vi "PrepRunDiluteExt_v01.vi"(2 "Debug Mode":bool, 3 "Elapsed Time(s)":dbl, 4 "State":enum16{"Edit", "Start", "Run", "End", "Idle"}(ring), 5 "Argument List In":string[](array[string])) -> (0 "Status Out":string, 1 "Argument List Out":string[](array[string]))   [LabVIEW 2011]
panel:
  in  "Pbub Prep":bool caption="Pre-run"
  out "Pbub Prep var":bool
  out "Pbub?":bool
  in  "Pbub Flow":dbl caption="P bubbler Flow (0-100 sccm)" format="%.2f"
  in  "Pbub Run":bool caption="Run"
  out "GAMFC3 var":dbl=100.0 caption="R3 (0-1000 sscm)" format="%.1f"
  out "GAMFC2 var":dbl=10.0 caption="R2 (0-100 sscm)" format="%.2f"
  out "GAMFC1 var":dbl caption="R1 (0-10 sscm)" format="%.2f"
  out "Ga Flow var":dbl caption="Ga Flow (0-10 sscm)" format="%.4f"
  out "In Prep var":bool
  out "Ga Prep var":bool
  out "Al Prep var":bool
  out "PH3 Prep var":bool
  out "AsH3 Prep var":bool
  out "prep_done":bool
  out "run started":bool
  out "first":bool=TRUE
  out "total time":dbl
  out "is OK?":bool
  out "AsH3?":bool
  out "PH3?":bool
  out "In?":bool
  out "Ga?":bool
  out "Al?":bool
  in  "AsH3 Prep":bool caption="Pre-run"
  in  "PH3 Prep":bool caption="Pre-run"
  in  "In Prep":bool caption="Pre-run"
  in  "prep_time":dbl caption="pre-run time (s)"
  in  "Al Prep":bool caption="Pre-run"
  in  "AsH3 Run":bool caption="Run"
  in  "AsH3 Flow":dbl caption="AsH3 Flow (0-10 sccm)" format="%.2f"
  in  "PH3 Flow":dbl caption="PH3 Flow (0-100 sccm)" format="%.2f"
  in  "PH3 Run":bool caption="Run"
  in  "In Flow":dbl caption="In Flow (0-100 sscm)" format="%.2f"
  in  "In Run":bool caption="Run"
  in  "Al Run":bool caption="Run"
  in  "Al Flow":dbl caption="Al Flow (0-100 sscm)" format="%.2f"
  in  "Cancel":bool
  in  "OK":bool
  out "tTotal(s) 2":dbl
  in  "Ga Tab Control":enum32{"Page 1", "Page 2", "Page 3"}(tab)
  in  "Ga Dilution":bool caption="Dilute"
  in  "Ga Run":bool caption="Run"
  in  "Ga Prep":bool caption="Pre-run"
  out "Ga Flow val":dbl=1.0 caption="Ga Flow (0-10 sscm)" format="%.4f"
  in  "Ga Flow set":dbl caption="Ga Flow (0-10 sscm)" format="%.4f"
  out "GAMFC1 val":dbl caption="R1 (0-10 sscm)" format="%.4f"
  out "GAMFC3 val":dbl=100.0 caption="R3 (0-1000 sscm)" format="%.1f"
  out "GAMFC2 val":dbl=10.0 caption="R2 (0-100 sscm)" format="%.2f"
  in  "GAMFC1 set":dbl=1.0 caption="R1 (0-10 sscm)" format="%.2f"
  in  "GAMFC2 set":dbl=10.0 caption="R2 (0-100 sscm)" format="%.2f"
  in  "GAMFC3 set":dbl=100.0 caption="R3 (0-1000 sscm)" format="%.1f"
  in  "Ga Calculated":u16(ring)=1 caption="Calculated" items=["Ga flow", "MFC1", "MFC2", "MFC3"]
  # "Add pre-run time to run time in editor."
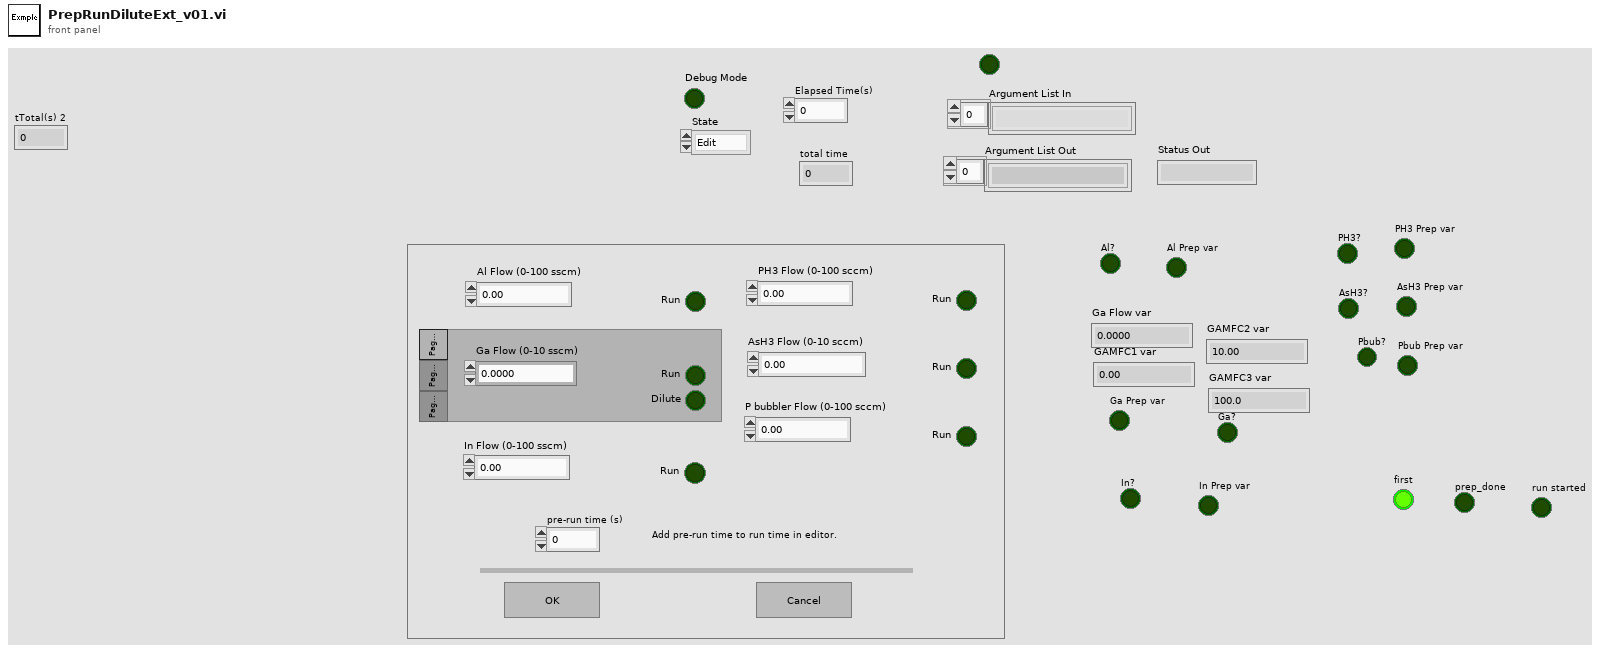
[diagram p1: front panel]
types:
  T1 = enum16{"Discrete", "Continuous", "Instantaneous", "Finite"}
  T2 = enum32{"Invalid", "Default", "Floating", "Floating/Auto-Hide", "Modal"}
  T3 = cluster{"Ga val":bool, "MFC1 val":bool, "MFC2 val":bool, "MFC3 val":bool, "Ga set":bool, "MFC1 set":bool, "MFC2 set":bool, "MFC3 set":bool}
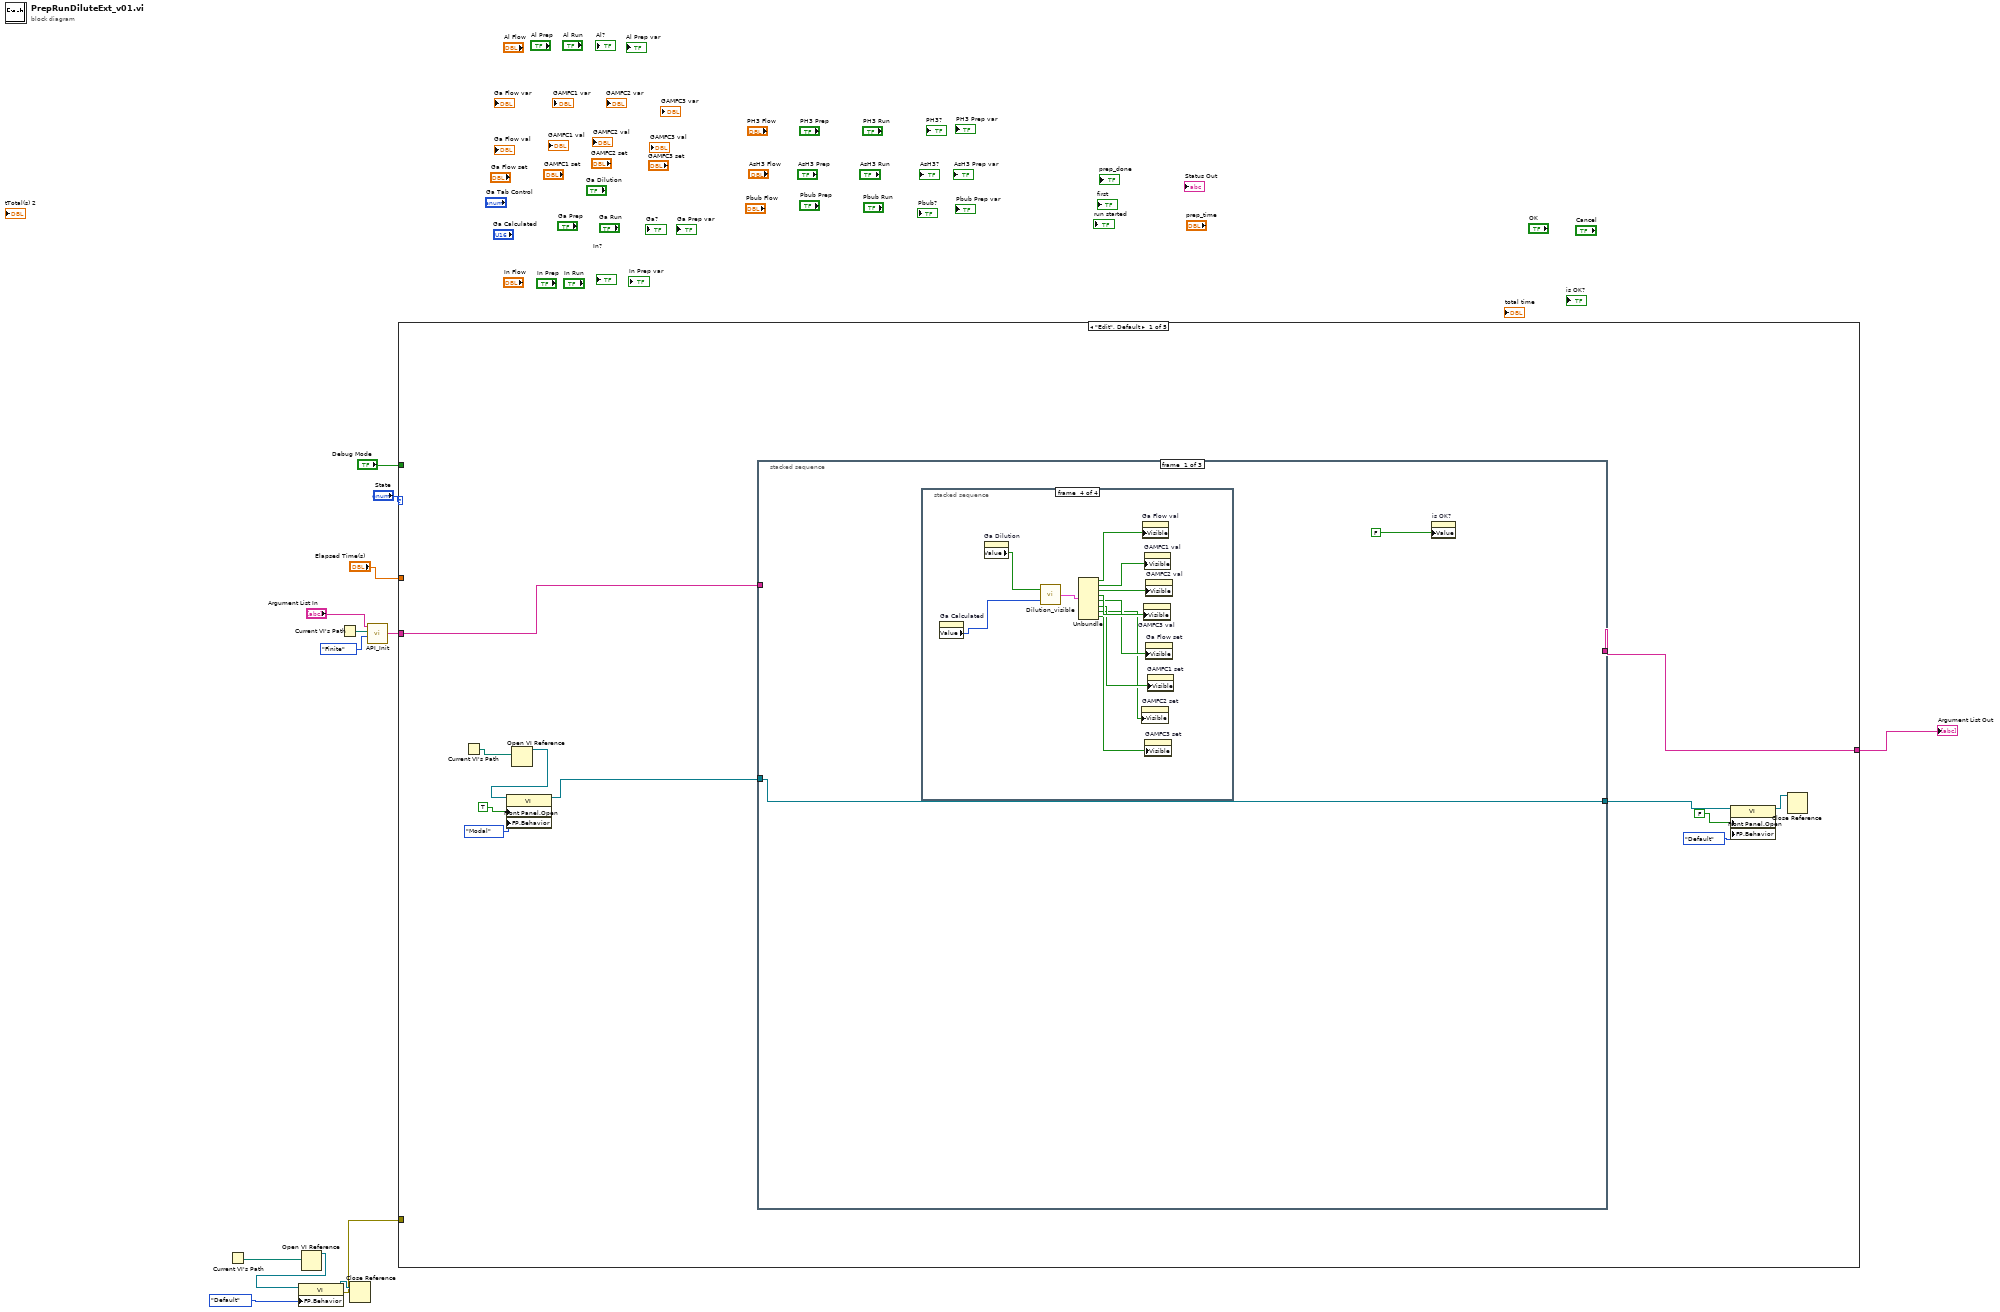
[diagram p0: block diagram]
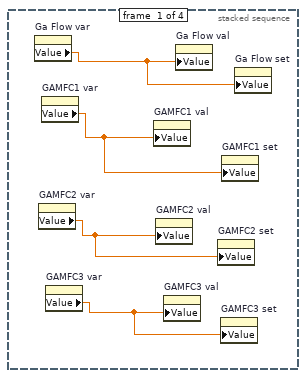
[diagram p2: hidden frame]
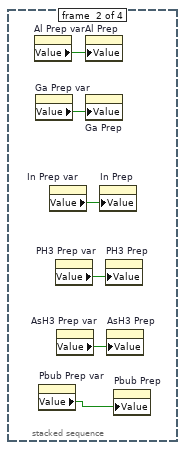
[diagram p3: hidden frame]
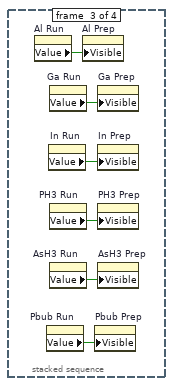
[diagram p4: hidden frame]
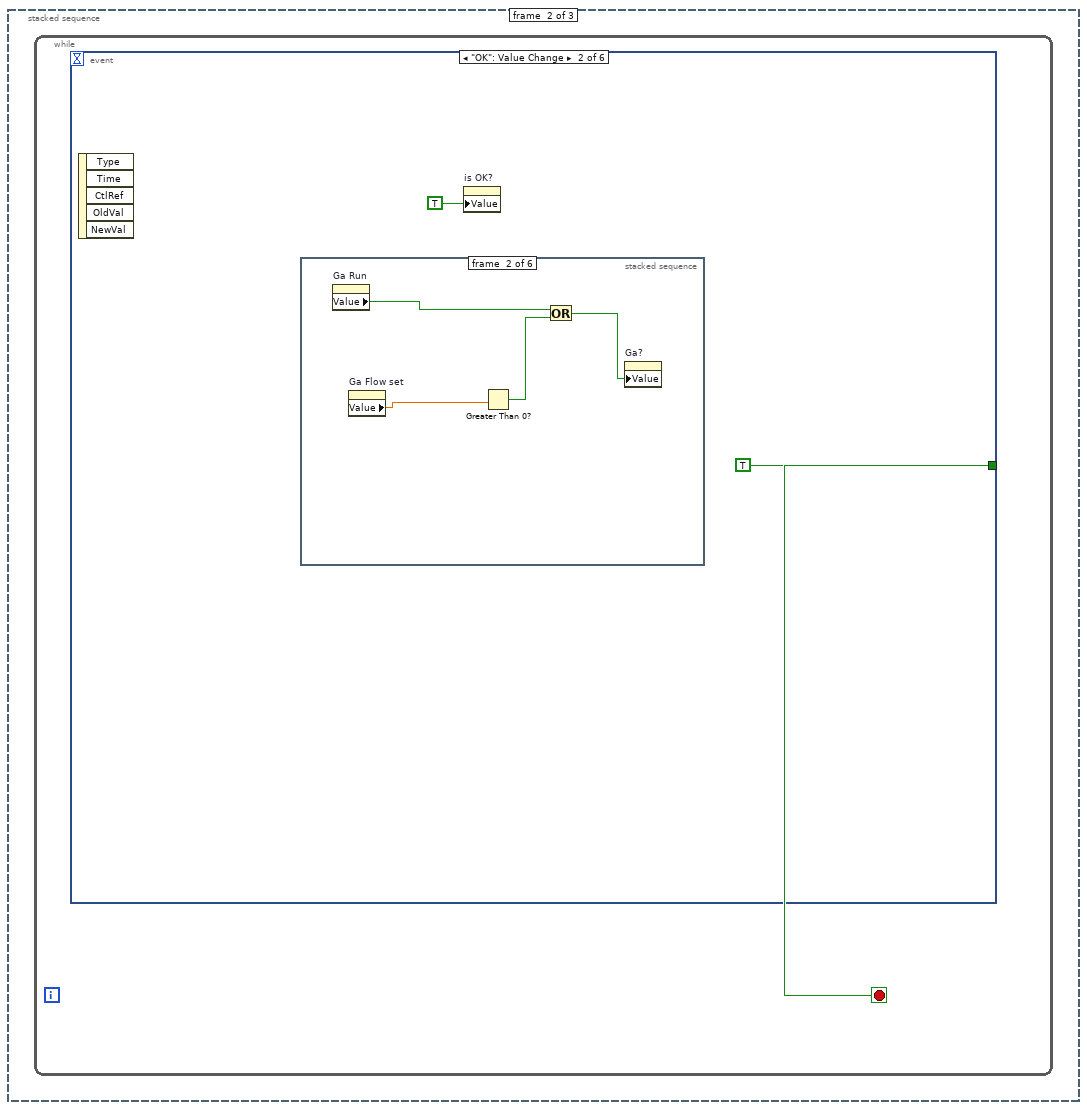
[diagram p5: hidden frame]
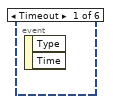
[diagram p6: hidden frame]
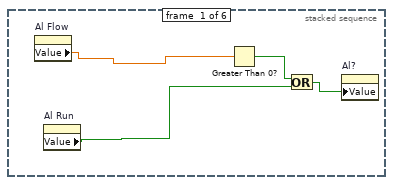
[diagram p7: hidden frame]
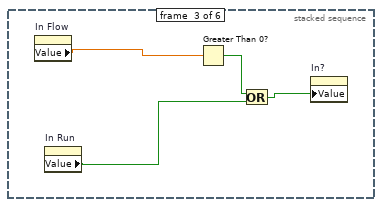
[diagram p8: hidden frame]
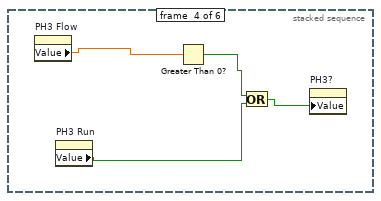
[diagram p9: hidden frame]
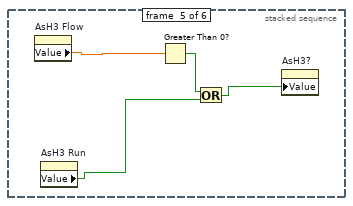
[diagram p10: hidden frame]
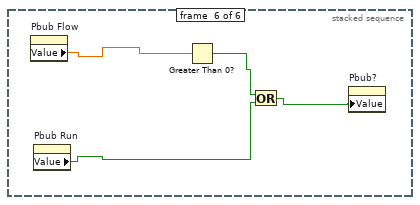
[diagram p11: hidden frame]
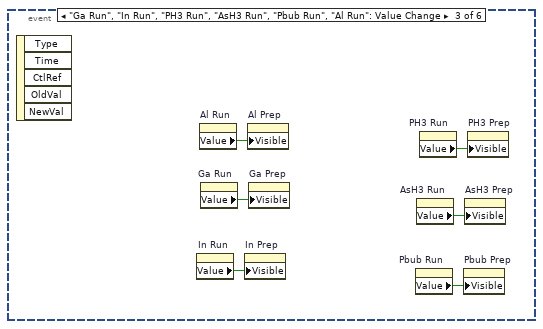
[diagram p12: hidden frame]
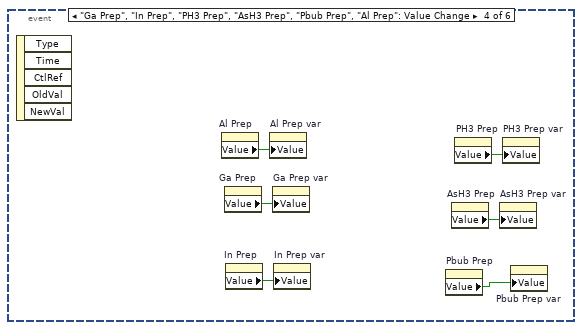
[diagram p13: hidden frame]
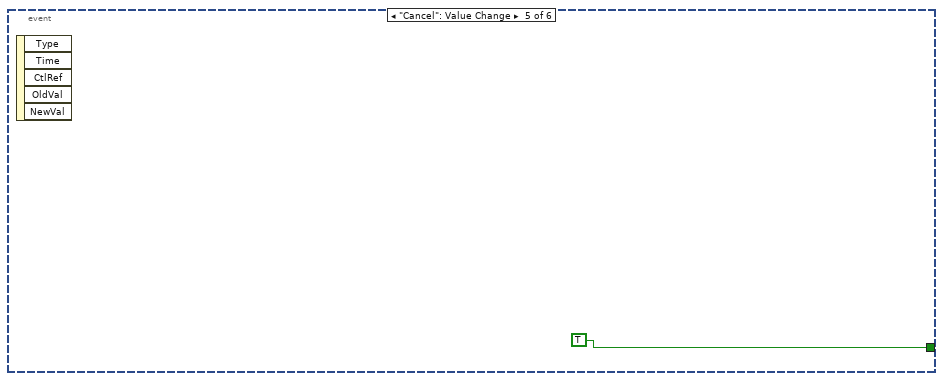
[diagram p14: hidden frame]
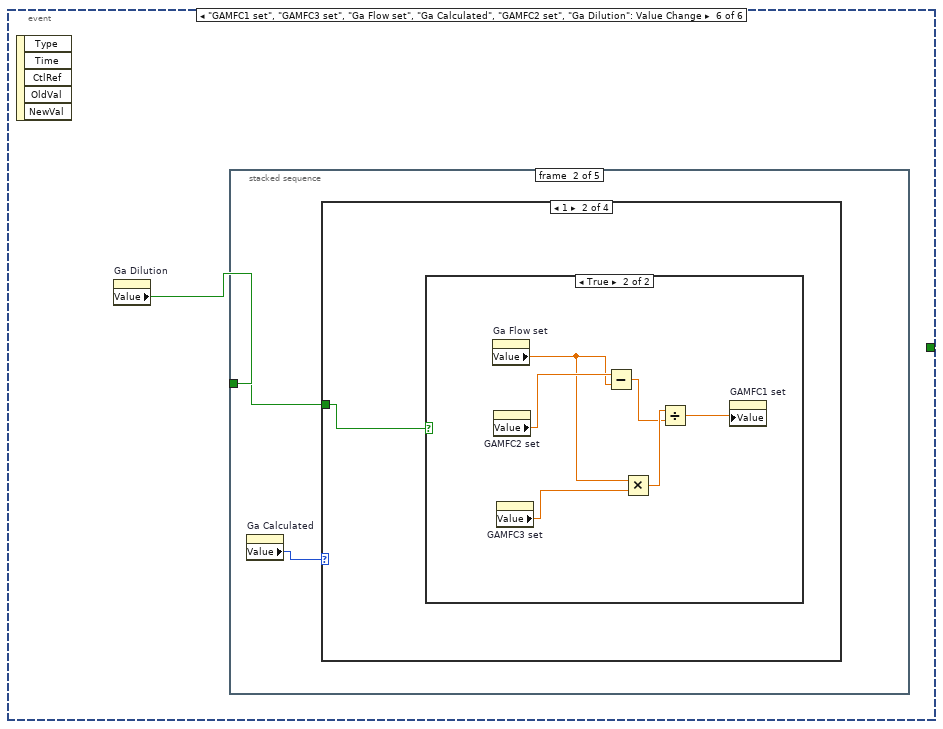
[diagram p15: hidden frame]
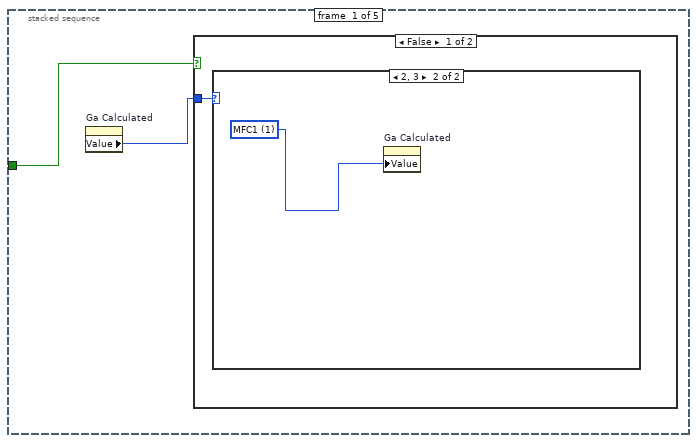
[diagram p16: hidden frame]
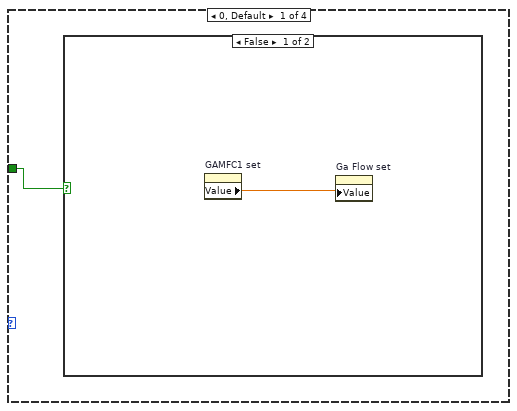
[diagram p19: hidden frame]
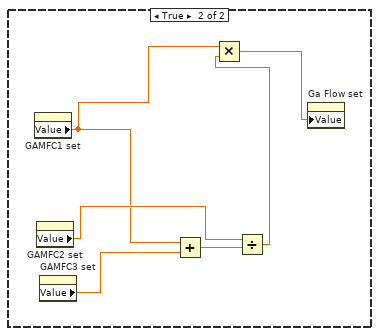
[diagram p20: hidden frame]
diagram:
  n1 = Current VI's Path() -> (path=w9:path)
  n2 = Open VI Reference(vi path=w9) -> (vi reference=w8:refnum<vi>)  [unwired: 1 in, 5 out]
  n3 = property class="VI"(reference=w8, "FP.Behavior"=T2."Default" ("Front Panel Window:Behavior")) -> (reference out=w6:refnum<vi>, error out=w5:errorcluster)  [unwired: 1 in]
  n4 = Current VI's Path() -> (path=w4:path)
  n5 = Close Reference(reference=w6) -> ()  [unwired: 1 in, 1 out]
  n6 = call "API_Init.vi"("API Mode"=T1."Finite", "VI Path"=w4, "Argument List In"="Argument List In") -> ("Argument List Out"=w1:string[])  [unwired: 1 in]
  n7 = case shown="\"Edit\", Default" "State" {
    tunnel: "Debug Mode" -> [_ w157 w222 _ _]
    tunnel: "Elapsed Time(s)" -> [_ _ w224 _ _]
    tunnel: w1 -> [w15 w159 w221 w355 w356]
    tunnel: [w14 w158 w223 w355 w356] -> w10
    tunnel: w5 -> [_ _ _ _ _]
    frame "Edit", Default {
      n8 = Current VI's Path() -> (path=w20:path)
      n9 = Open VI Reference(vi path=w20) -> (vi reference=w19:refnum<vi>)  [unwired: 1 in, 5 out]
      n10 = property class="VI"(reference=w19, "Front Panel.Open"=TRUE ("Front Panel Window:Open"), "FP.Behavior"=T2."Modal" ("Front Panel Window:Behavior")) -> (reference out=w18:refnum<vi>)  [unwired: 1 in, 1 out]
      n11 = stacked-sequence {
        tunnel: w15 -> [_ _ w152]
        tunnel: w18 -> [w26 _ _]
        tunnel: [w26 _ _] -> w22
        tunnel: [_ _ w150] -> w14
        frame #0 {
          n12 = stacked-sequence {
            frame #0 {
              n13 = property on="Ga Flow var" class="DigNum (strict)"() -> ("Value"=w30:dbl)  [unwired: 2 in, 2 out]
              n14 = property on="GAMFC2 var" class="DigNum (strict)"() -> ("Value"=w28:dbl)  [unwired: 2 in, 2 out]
              n15 = property on="GAMFC1 var" class="DigNum (strict)"() -> ("Value"=w27:dbl)  [unwired: 2 in, 2 out]
              n16 = property on="GAMFC3 var" class="DigNum (strict)"() -> ("Value"=w29:dbl)  [unwired: 2 in, 2 out]
              n17 = property on="GAMFC1 val" class="DigNum (strict)"("Value"=w27) -> ()  [unwired: 2 in, 2 out]
              n18 = property on="GAMFC2 val" class="DigNum (strict)"("Value"=w28) -> ()  [unwired: 2 in, 2 out]
              n19 = property on="GAMFC3 val" class="DigNum (strict)"("Value"=w29) -> ()  [unwired: 2 in, 2 out]
              n20 = property on="Ga Flow val" class="DigNum (strict)"("Value"=w30) -> ()  [unwired: 2 in, 2 out]
              n21 = property on="GAMFC2 set" class="DigNum (strict)"("Value"=w28) -> ()  [unwired: 2 in, 2 out]
              n22 = property on="GAMFC3 set" class="DigNum (strict)"("Value"=w29) -> ()  [unwired: 2 in, 2 out]
              n23 = property on="GAMFC1 set" class="DigNum (strict)"("Value"=w27) -> ()  [unwired: 2 in, 2 out]
              n24 = property on="Ga Flow set" class="DigNum (strict)"("Value"=w30) -> ()  [unwired: 2 in, 2 out]
            }
            frame #1 {
              n25 = property on="Al Prep var" class="Bool (strict)"() -> ("Value"=w36:bool)  [unwired: 2 in, 2 out]
              n26 = property on="Ga Prep var" class="Bool (strict)"() -> ("Value"=w35:bool)  [unwired: 2 in, 2 out]
              n27 = property on="Pbub Prep var" class="Bool (strict)"() -> ("Value"=w31:bool)  [unwired: 2 in, 2 out]
              n28 = property on="In Prep var" class="Bool (strict)"() -> ("Value"=w34:bool)  [unwired: 2 in, 2 out]
              n29 = property on="PH3 Prep var" class="Bool (strict)"() -> ("Value"=w33:bool)  [unwired: 2 in, 2 out]
              n30 = property on="AsH3 Prep var" class="Bool (strict)"() -> ("Value"=w32:bool)  [unwired: 2 in, 2 out]
              n31 = property on="Al Prep" class="Bool (strict)"("Value"=w36) -> ()  [unwired: 2 in, 2 out]
              n32 = property on="Ga Prep" class="Bool (strict)"("Value"=w35) -> ()  [unwired: 2 in, 2 out]
              n33 = property on="In Prep" class="Bool (strict)"("Value"=w34) -> ()  [unwired: 2 in, 2 out]
              n34 = property on="PH3 Prep" class="Bool (strict)"("Value"=w33) -> ()  [unwired: 2 in, 2 out]
              n35 = property on="AsH3 Prep" class="Bool (strict)"("Value"=w32) -> ()  [unwired: 2 in, 2 out]
              n36 = property on="Pbub Prep" class="Bool (strict)"("Value"=w31) -> ()  [unwired: 2 in, 2 out]
            }
            frame #2 {
              n37 = property on="Al Run" class="Bool (strict)"() -> ("Value"=w42:bool)  [unwired: 2 in, 2 out]
              n38 = property on="Pbub Run" class="Bool (strict)"() -> ("Value"=w37:bool)  [unwired: 2 in, 2 out]
              n39 = property on="In Run" class="Bool (strict)"() -> ("Value"=w40:bool)  [unwired: 2 in, 2 out]
              n40 = property on="Ga Run" class="Bool (strict)"() -> ("Value"=w41:bool)  [unwired: 2 in, 2 out]
              n41 = property on="PH3 Run" class="Bool (strict)"() -> ("Value"=w39:bool)  [unwired: 2 in, 2 out]
              n42 = property on="AsH3 Run" class="Bool (strict)"() -> ("Value"=w38:bool)  [unwired: 2 in, 2 out]
              n43 = property on="Al Prep" class="Bool (strict)"("Visible"=w42) -> ()  [unwired: 2 in, 2 out]
              n44 = property on="Pbub Prep" class="Bool (strict)"("Visible"=w37) -> ()  [unwired: 2 in, 2 out]
              n45 = property on="Ga Prep" class="Bool (strict)"("Visible"=w41) -> ()  [unwired: 2 in, 2 out]
              n46 = property on="In Prep" class="Bool (strict)"("Visible"=w40) -> ()  [unwired: 2 in, 2 out]
              n47 = property on="PH3 Prep" class="Bool (strict)"("Visible"=w39) -> ()  [unwired: 2 in, 2 out]
              n48 = property on="AsH3 Prep" class="Bool (strict)"("Visible"=w38) -> ()  [unwired: 2 in, 2 out]
            }
            frame #3 {
              n49 = property on="Ga Calculated" class="Ring (strict)"() -> ("Value"=w51:u16)  [unwired: 2 in, 2 out]
              n50 = property on="Ga Dilution" class="Bool (strict)"() -> ("Value"=w53:bool)  [unwired: 2 in, 2 out]
              n51 = call "Dilution_visible.vi"("calculated"=w51, "dilution"=w53) -> ("Visible"=w52:T3)
              n52 = Unbundle(w52) -> ("Ga val"=w50:bool, "MFC1 val"=w49:bool, "MFC2 val"=w48:bool, "MFC3 val"=w47:bool, "Ga set"=w46:bool, "MFC1 set"=w45:bool, "MFC2 set"=w44:bool, "MFC3 set"=w43:bool)
              n53 = property on="GAMFC2 set" class="DigNum (strict)"("Visible"=w44) -> ()  [unwired: 2 in, 2 out]
              n54 = property on="Ga Flow val" class="DigNum (strict)"("Visible"=w50) -> ()  [unwired: 2 in, 2 out]
              n55 = property on="GAMFC3 val" class="DigNum (strict)"("Visible"=w47) -> ()  [unwired: 2 in, 2 out]
              n56 = property on="GAMFC1 val" class="DigNum (strict)"("Visible"=w49) -> ()  [unwired: 2 in, 2 out]
              n57 = property on="GAMFC3 set" class="DigNum (strict)"("Visible"=w43) -> ()  [unwired: 2 in, 2 out]
              n58 = property on="GAMFC2 val" class="DigNum (strict)"("Visible"=w48) -> ()  [unwired: 2 in, 2 out]
              n59 = property on="Ga Flow set" class="DigNum (strict)"("Visible"=w46) -> ()  [unwired: 2 in, 2 out]
              n60 = property on="GAMFC1 set" class="DigNum (strict)"("Visible"=w45) -> ()  [unwired: 2 in, 2 out]
            }
          }
          n61 = property on="is OK?" class="Bool (strict)"("Value"=FALSE ("is OK?")) -> ()  [unwired: 2 in, 2 out]
        }
        frame #1 {
          n62 = while {
            stop <- w54 stop-if-true
            n63 = event shown="[1] \"OK\": Value Change" {
              selector: _ -> [_ _ _ _ _ _]
              dyn-events: _ -> [_ _ _ _ _ _]
              timeout: _ -> [_ _ _ _ _ _]
              tunnel: [_ TRUE _ _ TRUE _] -> w54
              event Timeout {
                n64 = event-data() -> ()  [unwired: 1 in, 2 out]
              }
              event "OK": Value Change {
                n65 = event-data() -> ()  [unwired: 1 in, 5 out]
                n66 = stacked-sequence {
                  frame #0 {
                    n67 = property on="Al Flow" class="DigNum (strict)"() -> ("Value"=w59:dbl)  [unwired: 2 in, 2 out]
                    n68 = property on="Al Run" class="Bool (strict)"() -> ("Value"=w58:bool)  [unwired: 2 in, 2 out]
                    n69 = Greater Than 0?(x=w59) -> (x > 0?=w60:bool)
                    n70 = Or(x=w60, y=w58) -> (x .or. y?=w57:bool)
                    n71 = property on="Al?" class="Bool (strict)"("Value"=w57) -> ()  [unwired: 2 in, 2 out]
                  }
                  frame #1 {
                    n72 = property on="Ga Run" class="Bool (strict)"() -> ("Value"=w62:bool)  [unwired: 2 in, 2 out]
                    n73 = property on="Ga Flow set" class="DigNum (strict)"() -> ("Value"=w63:dbl)  [unwired: 2 in, 2 out]
                    n74 = Greater Than 0?(x=w63) -> (x > 0?=w64:bool)
                    n75 = Or(x=w62, y=w64) -> (x .or. y?=w61:bool)
                    n76 = property on="Ga?" class="Bool (strict)"("Value"=w61) -> ()  [unwired: 2 in, 2 out]
                  }
                  frame #2 {
                    n77 = property on="In Flow" class="DigNum (strict)"() -> ("Value"=w66:dbl)  [unwired: 2 in, 2 out]
                    n78 = property on="In Run" class="Bool (strict)"() -> ("Value"=w67:bool)  [unwired: 2 in, 2 out]
                    n79 = Greater Than 0?(x=w66) -> (x > 0?=w68:bool)
                    n80 = Or(x=w68, y=w67) -> (x .or. y?=w65:bool)
                    n81 = property on="In?" class="Bool (strict)"("Value"=w65) -> ()  [unwired: 2 in, 2 out]
                  }
                  frame #3 {
                    n82 = property on="PH3 Flow" class="DigNum (strict)"() -> ("Value"=w71:dbl)  [unwired: 2 in, 2 out]
                    n83 = property on="PH3 Run" class="Bool (strict)"() -> ("Value"=w70:bool)  [unwired: 2 in, 2 out]
                    n84 = Greater Than 0?(x=w71) -> (x > 0?=w72:bool)
                    n85 = Or(x=w72, y=w70) -> (x .or. y?=w69:bool)
                    n86 = property on="PH3?" class="Bool (strict)"("Value"=w69) -> ()  [unwired: 2 in, 2 out]
                  }
                  frame #4 {
                    n87 = property on="AsH3 Flow" class="DigNum (strict)"() -> ("Value"=w75:dbl)  [unwired: 2 in, 2 out]
                    n88 = property on="AsH3 Run" class="Bool (strict)"() -> ("Value"=w74:bool)  [unwired: 2 in, 2 out]
                    n89 = Greater Than 0?(x=w75) -> (x > 0?=w76:bool)
                    n90 = Or(x=w76, y=w74) -> (x .or. y?=w73:bool)
                    n91 = property on="AsH3?" class="Bool (strict)"("Value"=w73) -> ()  [unwired: 2 in, 2 out]
                  }
                  frame #5 {
                    n92 = property on="Pbub Flow" class="DigNum (strict)"() -> ("Value"=w78:dbl)  [unwired: 2 in, 2 out]
                    n93 = property on="Pbub Run" class="Bool (strict)"() -> ("Value"=w77:bool)  [unwired: 2 in, 2 out]
                    n94 = Greater Than 0?(x=w78) -> (x > 0?=w80:bool)
                    n95 = Or(x=w80, y=w77) -> (x .or. y?=w79:bool)
                    n96 = property on="Pbub?" class="Bool (strict)"("Value"=w79) -> ()  [unwired: 2 in, 2 out]
                  }
                }
                n97 = property on="is OK?" class="Bool (strict)"("Value"=TRUE ("is OK?")) -> ()  [unwired: 2 in, 2 out]
              }
              event "Ga Run", "In Run", "PH3 Run", "AsH3 Run", "Pbub Run", "Al Run": Value Change {
                n98 = event-data() -> ()  [unwired: 1 in, 5 out]
                n99 = property on="In Run" class="Bool (strict)"() -> ("Value"=w84:bool)  [unwired: 2 in, 2 out]
                n100 = property on="Al Run" class="Bool (strict)"() -> ("Value"=w86:bool)  [unwired: 2 in, 2 out]
                n101 = property on="Ga Run" class="Bool (strict)"() -> ("Value"=w85:bool)  [unwired: 2 in, 2 out]
                n102 = property on="In Prep" class="Bool (strict)"("Visible"=w84) -> ()  [unwired: 2 in, 2 out]
                n103 = property on="Al Prep" class="Bool (strict)"("Visible"=w86) -> ()  [unwired: 2 in, 2 out]
                n104 = property on="Ga Prep" class="Bool (strict)"("Visible"=w85) -> ()  [unwired: 2 in, 2 out]
                n105 = property on="Pbub Run" class="Bool (strict)"() -> ("Value"=w81:bool)  [unwired: 2 in, 2 out]
                n106 = property on="AsH3 Run" class="Bool (strict)"() -> ("Value"=w83:bool)  [unwired: 2 in, 2 out]
                n107 = property on="PH3 Run" class="Bool (strict)"() -> ("Value"=w82:bool)  [unwired: 2 in, 2 out]
                n108 = property on="Pbub Prep" class="Bool (strict)"("Visible"=w81) -> ()  [unwired: 2 in, 2 out]
                n109 = property on="AsH3 Prep" class="Bool (strict)"("Visible"=w83) -> ()  [unwired: 2 in, 2 out]
                n110 = property on="PH3 Prep" class="Bool (strict)"("Visible"=w82) -> ()  [unwired: 2 in, 2 out]
              }
              event "Ga Prep", "In Prep", "PH3 Prep", "AsH3 Prep", "Pbub Prep", "Al Prep": Value Change {
                n111 = event-data() -> ()  [unwired: 1 in, 5 out]
                n112 = property on="Al Prep" class="Bool (strict)"() -> ("Value"=w92:bool)  [unwired: 2 in, 2 out]
                n113 = property on="Ga Prep" class="Bool (strict)"() -> ("Value"=w91:bool)  [unwired: 2 in, 2 out]
                n114 = property on="In Prep" class="Bool (strict)"() -> ("Value"=w90:bool)  [unwired: 2 in, 2 out]
                n115 = property on="Al Prep var" class="Bool (strict)"("Value"=w92) -> ()  [unwired: 2 in, 2 out]
                n116 = property on="Ga Prep var" class="Bool (strict)"("Value"=w91) -> ()  [unwired: 2 in, 2 out]
                n117 = property on="In Prep var" class="Bool (strict)"("Value"=w90) -> ()  [unwired: 2 in, 2 out]
                n118 = property on="Pbub Prep" class="Bool (strict)"() -> ("Value"=w87:bool)  [unwired: 2 in, 2 out]
                n119 = property on="AsH3 Prep" class="Bool (strict)"() -> ("Value"=w88:bool)  [unwired: 2 in, 2 out]
                n120 = property on="PH3 Prep" class="Bool (strict)"() -> ("Value"=w89:bool)  [unwired: 2 in, 2 out]
                n121 = property on="AsH3 Prep var" class="Bool (strict)"("Value"=w88) -> ()  [unwired: 2 in, 2 out]
                n122 = property on="PH3 Prep var" class="Bool (strict)"("Value"=w89) -> ()  [unwired: 2 in, 2 out]
                n123 = property on="Pbub Prep var" class="Bool (strict)"("Value"=w87) -> ()  [unwired: 2 in, 2 out]
              }
              event "Cancel": Value Change {
                n124 = event-data() -> ()  [unwired: 1 in, 5 out]
              }
              event "GAMFC1 set", "GAMFC3 set", "Ga Flow set", "Ga Calculated", "GAMFC2 set", "Ga Dilution": Value Change {
                n125 = event-data() -> ()  [unwired: 1 in, 5 out]
                n126 = property on="Ga Dilution" class="Bool (strict)"() -> ("Value"=w94:bool)  [unwired: 2 in, 2 out]
                n127 = stacked-sequence {
                  tunnel: w94 -> [w96 w100 w141 _ w146]
                  frame #0 {
                    n128 = property on="Ga Calculated" class="Ring (strict)"() -> ("Value"=w95:u16)  [unwired: 2 in, 2 out]
                    n129 = case shown="False" w96 {
                      tunnel: w95 -> [w97 _]
                      frame False {
                        n130 = case shown="2, 3" w97 {
                          frame 0, 1, Default {
                          }
                          frame 2, 3 {
                            w98 = u16 1 items=["Ga flow", "MFC1", "MFC2", "MFC3"] ("Ga calculated")
                            n131 = property on="Ga Calculated" class="Ring (strict)"("Value"=w98) -> ()  [unwired: 2 in, 2 out]
                          }
                        }
                      }
                      frame True {
                      }
                    }
                  }
                  frame #1 {
                    n132 = property on="Ga Calculated" class="Ring (strict)"() -> ("Value"=w99:u16)  [unwired: 2 in, 2 out]
                    n133 = case shown="1" w99 {
                      tunnel: w100 -> [w101 w109 w117 w124]
                      frame 0, Default {
                        n134 = case shown="False" w101 {
                          frame False {
                            n135 = property on="GAMFC1 set" class="DigNum (strict)"() -> ("Value"=w102:dbl)  [unwired: 2 in, 2 out]
                            n136 = property on="Ga Flow set" class="DigNum (strict)"("Value"=w102) -> ()  [unwired: 2 in, 2 out]
                          }
                          frame True {
                            n137 = property on="GAMFC1 set" class="DigNum (strict)"() -> ("Value"=w104:dbl)  [unwired: 2 in, 2 out]
                            n138 = property on="GAMFC2 set" class="DigNum (strict)"() -> ("Value"=w106:dbl)  [unwired: 2 in, 2 out]
                            n139 = property on="GAMFC3 set" class="DigNum (strict)"() -> ("Value"=w108:dbl)  [unwired: 2 in, 2 out]
                            n140 = Add(x=w104, y=w108) -> (x+y=w107:dbl)
                            n141 = Divide(x=w106, y=w107) -> (x/y=w105:dbl)
                            n142 = Multiply(x=w104, y=w105) -> (x*y=w103:dbl)
                            n143 = property on="Ga Flow set" class="DigNum (strict)"("Value"=w103) -> ()  [unwired: 2 in, 2 out]
                          }
                        }
                      }
                      frame 1 {
                        n144 = case shown="True" w109 {
                          frame False {
                            n145 = property on="Ga Flow set" class="DigNum (strict)"() -> ("Value"=w110:dbl)  [unwired: 2 in, 2 out]
                            n146 = property on="GAMFC1 set" class="DigNum (strict)"("Value"=w110) -> ()  [unwired: 2 in, 2 out]
                          }
                          frame True {
                            n147 = property on="Ga Flow set" class="DigNum (strict)"() -> ("Value"=w115:dbl)  [unwired: 2 in, 2 out]
                            n148 = property on="GAMFC2 set" class="DigNum (strict)"() -> ("Value"=w116:dbl)  [unwired: 2 in, 2 out]
                            n149 = property on="GAMFC3 set" class="DigNum (strict)"() -> ("Value"=w114:dbl)  [unwired: 2 in, 2 out]
                            n150 = Subtract(x=w116, y=w115) -> (x-y=w112:dbl)
                            n151 = Multiply(x=w115, y=w114) -> (x*y=w113:dbl)
                            n152 = Divide(x=w113, y=w112) -> (x/y=w111:dbl)
                            n153 = property on="GAMFC1 set" class="DigNum (strict)"("Value"=w111) -> ()  [unwired: 2 in, 2 out]
                          }
                        }
                      }
                      frame 2 {
                        n154 = case shown="True" w117 {
                          frame False {
                          }
                          frame True {
                            n155 = property on="GAMFC1 set" class="DigNum (strict)"() -> ("Value"=w119:dbl)  [unwired: 2 in, 2 out]
                            n156 = property on="GAMFC3 set" class="DigNum (strict)"() -> ("Value"=w121:dbl)  [unwired: 2 in, 2 out]
                            n157 = property on="Ga Flow set" class="DigNum (strict)"() -> ("Value"=w122:dbl)  [unwired: 2 in, 2 out]
                            n158 = Add(x=w119, y=w121) -> (x+y=w123:dbl)
                            n159 = Multiply(x=w122, y=w123) -> (x*y=w120:dbl)
                            n160 = Divide(x=w120, y=w119) -> (x/y=w118:dbl)
                            n161 = property on="GAMFC2 set" class="DigNum (strict)"("Value"=w118) -> ()  [unwired: 2 in, 2 out]
                          }
                        }
                      }
                      frame 3 {
                        n162 = case shown="True" w124 {
                          frame False {
                          }
                          frame True {
                            n163 = property on="GAMFC2 set" class="DigNum (strict)"() -> ("Value"=w130:dbl)  [unwired: 2 in, 2 out]
                            n164 = property on="Ga Flow set" class="DigNum (strict)"() -> ("Value"=w128:dbl)  [unwired: 2 in, 2 out]
                            n165 = property on="GAMFC1 set" class="DigNum (strict)"() -> ("Value"=w129:dbl)  [unwired: 2 in, 2 out]
                            n166 = Subtract(x=w130, y=w128) -> (x-y=w126:dbl)
                            n167 = Divide(x=w129, y=w128) -> (x/y=w127:dbl)
                            n168 = Multiply(x=w127, y=w126) -> (x*y=w125:dbl)
                            n169 = property on="GAMFC3 set" class="DigNum (strict)"("Value"=w125) -> ()  [unwired: 2 in, 2 out]
                          }
                        }
                      }
                    }
                  }
                  frame #2 {
                    n170 = property on="Ga Calculated" class="Ring (strict)"() -> ("Value"=w131:u16)  [unwired: 2 in, 2 out]
                    n171 = call "Dilution_visible.vi"("calculated"=w131, "dilution"=w141) -> ("Visible"=w137:T3)
                    n172 = Unbundle(w137) -> ("Ga val"=w140:bool, "MFC1 val"=w139:bool, "MFC2 val"=w138:bool, "MFC3 val"=w136:bool, "Ga set"=w135:bool, "MFC1 set"=w134:bool, "MFC2 set"=w133:bool, "MFC3 set"=w132:bool)
                    n173 = property on="Ga Flow set" class="DigNum (strict)"("Visible"=w135) -> ()  [unwired: 2 in, 2 out]
                    n174 = property on="GAMFC1 set" class="DigNum (strict)"("Visible"=w134) -> ()  [unwired: 2 in, 2 out]
                    n175 = property on="GAMFC3 set" class="DigNum (strict)"("Visible"=w132) -> ()  [unwired: 2 in, 2 out]
                    n176 = property on="GAMFC2 set" class="DigNum (strict)"("Visible"=w133) -> ()  [unwired: 2 in, 2 out]
                    n177 = property on="Ga Flow val" class="DigNum (strict)"("Visible"=w140) -> ()  [unwired: 2 in, 2 out]
                    n178 = property on="GAMFC1 val" class="DigNum (strict)"("Visible"=w139) -> ()  [unwired: 2 in, 2 out]
                    n179 = property on="GAMFC2 val" class="DigNum (strict)"("Visible"=w138) -> ()  [unwired: 2 in, 2 out]
                    n180 = property on="GAMFC3 val" class="DigNum (strict)"("Visible"=w136) -> ()  [unwired: 2 in, 2 out]
                  }
                  frame #3 {
                    n181 = property on="GAMFC1 set" class="DigNum (strict)"() -> ("Value"=w144:dbl)  [unwired: 2 in, 2 out]
                    n182 = property on="Ga Flow set" class="DigNum (strict)"() -> ("Value"=w145:dbl)  [unwired: 2 in, 2 out]
                    n183 = property on="GAMFC2 set" class="DigNum (strict)"() -> ("Value"=w143:dbl)  [unwired: 2 in, 2 out]
                    n184 = property on="GAMFC3 set" class="DigNum (strict)"() -> ("Value"=w142:dbl)  [unwired: 2 in, 2 out]
                    n185 = property on="GAMFC3 val" class="DigNum (strict)"("Value"=w142) -> ()  [unwired: 2 in, 2 out]
                    n186 = property on="GAMFC1 val" class="DigNum (strict)"("Value"=w144) -> ()  [unwired: 2 in, 2 out]
                    n187 = property on="GAMFC2 val" class="DigNum (strict)"("Value"=w143) -> ()  [unwired: 2 in, 2 out]
                    n188 = property on="Ga Flow val" class="DigNum (strict)"("Value"=w145) -> ()  [unwired: 2 in, 2 out]
                    n189 = property on="GAMFC3 var" class="DigNum (strict)"("Value"=w142) -> ()  [unwired: 2 in, 2 out]
                    n190 = property on="GAMFC1 var" class="DigNum (strict)"("Value"=w144) -> ()  [unwired: 2 in, 2 out]
                    n191 = property on="GAMFC2 var" class="DigNum (strict)"("Value"=w143) -> ()  [unwired: 2 in, 2 out]
                    n192 = property on="Ga Flow var" class="DigNum (strict)"("Value"=w145) -> ()  [unwired: 2 in, 2 out]
                  }
                  frame #4 {
                    n193 = case shown="True" w146 {
                      frame False {
                        n194 = property on="Ga Calculated" class="Ring (strict)"("Disabled Items []"=i32[] [2, 3]) -> ()  [unwired: 2 in, 2 out]
                      }
                      frame True {
                        n195 = property on="Ga Calculated" class="Ring (strict)"("Disabled Items []"=i32[] []) -> ()  [unwired: 2 in, 2 out]
                      }
                    }
                  }
                }
              }
            }
          }
        }
        frame #2 {
          n196 = property on="is OK?" class="Bool (strict)"() -> ("Value"=w149:bool)  [unwired: 2 in, 2 out]
          n197 = case shown="True" w149 {
            tunnel: w152 -> [w155 w156]
            tunnel: [w155 w156] -> w151
            frame False {
            }
            frame True {
            }
          }
          n198 = Not(x=w149) -> (.not. x?=w154:bool)
          n199 = Current VI's Path() -> (path=w153:path)
          n200 = call "API_Edit.vi"("Cancel"=w154, "OK"=w149, "VI Path"=w153, "Argument List In"=w151) -> ("Argument List Out"=w150:string[])
        }
      }
      n201 = property class="VI"(reference=w22, "Front Panel.Open"=FALSE ("Front Panel Window:Open"), "FP.Behavior"=T2."Default" ("Front Panel Window:Behavior")) -> (reference out=w23:refnum<vi>)  [unwired: 1 in, 1 out]
      n202 = Close Reference(reference=w23) -> ()  [unwired: 1 in, 1 out]
    }
    frame "Start" {
      n203 = call "Set_Argument.vi"("Enable"=FALSE, "Argument"="run_started", "Argument List In"=w159) -> ("Argument List Out"=w158:string[])
      n204 = stacked-sequence {
        tunnel: w157 -> [w162 w171 w183 w192 w202 w212]
        frame #0 {
          n205 = case shown="False" w162 {
            frame False {
              n206 = property on="Al?" class="Bool (strict)"() -> ("Value"=w163:bool)  [unwired: 2 in, 2 out]
              n207 = case shown="True" w163 {
                frame False {
                  w164 = FALSE ("Al Active")
                  n208 = call "set_Al.vi"("ALMFC1"=0.0 ("Aluminum Flow"), "Remote"=w164, "Run"=w164, "Bubbler In"=w164, "Active"=w164) -> ()  [unwired: 5 out]
                }
                frame True {
                  w170 = TRUE ("Al Active")
                  n209 = property on="Al Prep" class="Bool (strict)"() -> ("Value"=w168:bool)  [unwired: 2 in, 2 out]
                  n210 = property on="Al Run" class="Bool (strict)"() -> ("Value"=w167:bool)  [unwired: 2 in, 2 out]
                  n211 = property on="Al Flow" class="DigNum (strict)"() -> ("Value"=w169:dbl)  [unwired: 2 in, 2 out]
                  n212 = And(x=w168, y=w167) -> (x .and. y?=w166:bool)
                  n213 = call "set_Al.vi"("ALMFC1"=w169, "Run"=w166, "Bubbler In"=w170, "Active"=w170) -> ()  [unwired: 1 in, 5 out]
                }
              }
            }
            frame True {
            }
          }
        }
        frame #1 {
          n214 = case shown="False" w171 {
            frame False {
              n215 = property on="Ga?" class="Bool (strict)"() -> ("Value"=w172:bool)  [unwired: 2 in, 2 out]
              n216 = case shown="True" w172 {
                frame False {
                  w174 = FALSE ("Ga Active")
                  w173 = 0.0 ("Ga Flow 1")
                  n217 = call "set_Ga.vi"("Active"=w174, "GAMFC3"=w173, "GAMFC2"=w173, "GAMFC1"=w173, "Bubbler In"=w174, "H2 Dilute"=w174, "Run"=w174, "Remote"=w174) -> ()  [unwired: 8 out]
                }
                frame True {
                  w178 = TRUE ("Ga Active")
                  n218 = property on="GAMFC3 var" class="DigNum (strict)"() -> ("Value"=w175:dbl)  [unwired: 2 in, 2 out]
                  n219 = property on="GAMFC2 var" class="DigNum (strict)"() -> ("Value"=w176:dbl)  [unwired: 2 in, 2 out]
                  n220 = property on="GAMFC1 var" class="DigNum (strict)"() -> ("Value"=w177:dbl)  [unwired: 2 in, 2 out]
                  n221 = property on="Ga Prep var" class="Bool (strict)"() -> ("Value"=w179:bool)  [unwired: 2 in, 2 out]
                  n222 = property on="Ga Run" class="Bool (strict)"() -> ("Value"=w180:bool)  [unwired: 2 in, 2 out]
                  n223 = And(x=w179, y=w180) -> (x .and. y?=w182:bool)
                  n224 = property on="Ga Dilution" class="Bool (strict)"() -> ("Value"=w181:bool)  [unwired: 2 in, 2 out]
                  n225 = call "set_Ga.vi"("Active"=w178, "GAMFC3"=w175, "GAMFC2"=w176, "GAMFC1"=w177, "Bubbler In"=w178, "H2 Dilute"=w181, "Run"=w182, "Remote"=w178) -> ()  [unwired: 8 in]
                }
              }
            }
            frame True {
            }
          }
        }
        frame #2 {
          n226 = case shown="False" w183 {
            frame False {
              n227 = property on="In?" class="Bool (strict)"() -> ("Value"=w184:bool)  [unwired: 2 in, 2 out]
              n228 = case shown="True" w184 {
                frame False {
                  w186 = FALSE ("In Remote")
                  n229 = call "set_In.vi"("INMFC1"=0.0 ("Indium Flow"), "Remote"=w186, "Run"=w186, "Bubbler In"=w186, "Active"=w186) -> ()  [unwired: 5 out]
                }
                frame True {
                  w191 = TRUE ("In Run")
                  n230 = property on="In Run" class="Bool (strict)"() -> ("Value"=w188:bool)  [unwired: 2 in, 2 out]
                  n231 = property on="In Prep" class="Bool (strict)"() -> ("Value"=w189:bool)  [unwired: 2 in, 2 out]
                  n232 = And(x=w189, y=w188) -> (x .and. y?=w187:bool)
                  n233 = property on="In Flow" class="DigNum (strict)"() -> ("Value"=w190:dbl)  [unwired: 2 in, 2 out]
                  n234 = call "set_In.vi"("INMFC1"=w190, "Run"=w187, "Bubbler In"=w191, "Active"=w191) -> ()  [unwired: 1 in, 5 out]
                }
              }
            }
            frame True {
            }
          }
        }
        frame #3 {
          n235 = case shown="False" w192 {
            frame False {
              n236 = property on="PH3?" class="Bool (strict)"() -> ("Value"=w193:bool)  [unwired: 2 in, 2 out]
              n237 = case shown="False" w193 {
                frame False {
                  w194 = FALSE ("P_Gas Active")
                  n238 = call "set_P_gas.vi"("Run"=w194, "Gas In"=w194, "Active"=w194, "P_Gas Remote"=w194, "H2 Flush"=w194, "P_Gas Flow"=0.0) -> ()
                }
                frame True {
                  w197 = TRUE ("P_Gas Active")
                  n239 = property on="PH3 Flow" class="DigNum (strict)"() -> ("Value"=w201:dbl)  [unwired: 2 in, 2 out]
                  n240 = property on="PH3 Prep" class="Bool (strict)"() -> ("Value"=w200:bool)  [unwired: 2 in, 2 out]
                  n241 = property on="PH3 Run" class="Bool (strict)"() -> ("Value"=w199:bool)  [unwired: 2 in, 2 out]
                  n242 = And(x=w200, y=w199) -> (x .and. y?=w198:bool)
                  n243 = call "set_P_gas.vi"("Run"=w197, "Gas In"=w197, "Active"=w197, "P_Gas Remote"=w198, "H2 Flush"=FALSE, "P_Gas Flow"=w201) -> ()
                }
              }
            }
            frame True {
            }
          }
        }
        frame #4 {
          n244 = case shown="False" w202 {
            frame False {
              n245 = property on="AsH3?" class="Bool (strict)"() -> ("Value"=w203:bool)  [unwired: 2 in, 2 out]
              n246 = case shown="True" w203 {
                frame False {
                  w204 = FALSE ("As_Gas Active")
                  n247 = call "set_As_gas.vi"("Active"=w204, "As_Gas Flow"=0.0, "Gas In"=w204, "H2 Flush"=w204, "Run"=w204, "Remote"=w204) -> ()  [unwired: 10 in]
                }
                frame True {
                  w211 = TRUE ("As_Gas Active")
                  n248 = property on="AsH3 Prep" class="Bool (strict)"() -> ("Value"=w208:bool)  [unwired: 2 in, 2 out]
                  n249 = property on="AsH3 Run" class="Bool (strict)"() -> ("Value"=w209:bool)  [unwired: 2 in, 2 out]
                  n250 = property on="AsH3 Flow" class="DigNum (strict)"() -> ("Value"=w210:dbl)  [unwired: 2 in, 2 out]
                  n251 = And(x=w208, y=w209) -> (x .and. y?=w207:bool)
                  n252 = call "set_As_gas.vi"("Active"=w211, "As_Gas Flow"=w210, "Gas In"=w211, "H2 Flush"=FALSE, "Run"=w207) -> ()  [unwired: 11 in]
                }
              }
            }
            frame True {
            }
          }
        }
        frame #5 {
          n253 = case shown="False" w212 {
            frame False {
              n254 = property on="Pbub?" class="Bool (strict)"() -> ("Value"=w213:bool)  [unwired: 2 in, 2 out]
              n255 = case shown="True" w213 {
                frame False {
                  w215 = FALSE ("P_Liq Active")
                  n256 = call "set_In.vi"("INMFC1"=0.0 ("P_Liq Flow"), "Remote"=w215, "Run"=w215, "Bubbler In"=w215, "Active"=w215) -> ()  [unwired: 5 in]
                }
                frame True {
                  w216 = TRUE ("P_Liq Bubbler")
                  n257 = property on="Pbub Run" class="Bool (strict)"() -> ("Value"=w219:bool)  [unwired: 2 in, 2 out]
                  n258 = property on="Pbub Prep" class="Bool (strict)"() -> ("Value"=w220:bool)  [unwired: 2 in, 2 out]
                  n259 = property on="Pbub Flow" class="DigNum (strict)"() -> ("Value"=w218:dbl)  [unwired: 2 in, 2 out]
                  n260 = And(x=w220, y=w219) -> (x .and. y?=w217:bool)
                  n261 = call "set_P_Liq.vi"("flow 1"=w218, "Run"=w217, "Bubbler In"=w216, "Active"=w216) -> ()  [unwired: 6 in]
                }
              }
            }
            frame True {
            }
          }
        }
      }
    }
    frame "Run" {
      n262 = stacked-sequence {
        tunnel: w224 -> [_ w229 _ _]
        tunnel: w221 -> [w226 _ _ w292]
        tunnel: [_ _ _ w291] -> w223
        tunnel: w222 -> [_ _ _ w293]
        frame #0 {
          n263 = call "Get_Argument.vi"("Argument"="run_started", "Argument List"=w226) -> ("Enabled"=w225:bool)
          n264 = local write "run started"(w225) -> ()
        }
        frame #1 {
          n265 = property on="prep_time" class="DigNum (strict)"() -> ("Value"=w230:dbl)  [unwired: 2 in, 2 out]
          n266 = Greater Or Equal?(x=w229, y=w230) -> (x >= y?=w228:bool)
          n267 = local write "prep_done"(w228) -> ()
        }
        frame #2 {
          n268 = local read "run started"() -> (w232:bool)
          n269 = Not(x=w232) -> (.not. x?=w231:bool)
          n270 = stacked-sequence {
            tunnel: w231 -> [w234 w238 w247 w256 w265 w274 w285]
            frame #0 {
              n271 = case shown="True" w234 {
                tunnel: ["run: " "pre-run: "] -> w233
                frame False {
                }
                frame True {
                }
              }
              n272 = property on="Status Out" class="Str"("Value"=w233) -> ()  [unwired: 2 in, 2 out]
            }
            frame #1 {
              n273 = property on="Status Out" class="Str"() -> ("Value"=w244:string)  [unwired: 2 in, 2 out]
              n274 = property on="Al?" class="Bool (strict)"() -> ("Value"=w245:bool)  [unwired: 2 in, 2 out]
              n275 = property on="Al Run" class="Bool (strict)"() -> ("Value"=w237:bool)  [unwired: 2 in, 2 out]
              n276 = property on="Al Prep" class="Bool (strict)"() -> ("Value"=w239:bool)  [unwired: 2 in, 2 out]
              n277 = call "flow_strings.vi"("string in"=w244, "is first in?"=TRUE, "use source?"=w245, "name"="Al", "run source?"=w237, "prep source?"=w239, "is prep?"=w238) -> ("string out"=w243:string, "is first out?"=w242:bool)
              n278 = property on="Status Out" class="Str"("Value"=w243) -> ()  [unwired: 2 in, 2 out]
              n279 = property on="first" class="Bool (strict)"("Value"=w242) -> ()  [unwired: 2 in, 2 out]
            }
            frame #2 {
              n280 = property on="first" class="Bool (strict)"() -> ("Value"=w250:bool)  [unwired: 2 in, 2 out]
              n281 = property on="Status Out" class="Str"() -> ("Value"=w253:string)  [unwired: 2 in, 2 out]
              n282 = property on="Ga?" class="Bool (strict)"() -> ("Value"=w251:bool)  [unwired: 2 in, 2 out]
              n283 = property on="Ga Run" class="Bool (strict)"() -> ("Value"=w246:bool)  [unwired: 2 in, 2 out]
              n284 = property on="Ga Prep" class="Bool (strict)"() -> ("Value"=w248:bool)  [unwired: 2 in, 2 out]
              n285 = call "flow_strings.vi"("string in"=w253, "is first in?"=w250, "use source?"=w251, "name"="Ga", "run source?"=w246, "prep source?"=w248, "is prep?"=w247) -> ("string out"=w254:string, "is first out?"=w249:bool)
              n286 = property on="Status Out" class="Str"("Value"=w254) -> ()  [unwired: 2 in, 2 out]
              n287 = property on="first" class="Bool (strict)"("Value"=w249) -> ()  [unwired: 2 in, 2 out]
            }
            frame #3 {
              n288 = property on="first" class="Bool (strict)"() -> ("Value"=w260:bool)  [unwired: 2 in, 2 out]
              n289 = property on="Status Out" class="Str"() -> ("Value"=w262:string)  [unwired: 2 in, 2 out]
              n290 = property on="In?" class="Bool (strict)"() -> ("Value"=w263:bool)  [unwired: 2 in, 2 out]
              n291 = property on="In Run" class="Bool (strict)"() -> ("Value"=w255:bool)  [unwired: 2 in, 2 out]
              n292 = property on="In Prep" class="Bool (strict)"() -> ("Value"=w257:bool)  [unwired: 2 in, 2 out]
              n293 = call "flow_strings.vi"("string in"=w262, "is first in?"=w260, "use source?"=w263, "name"="In", "run source?"=w255, "prep source?"=w257, "is prep?"=w256) -> ("string out"=w259:string, "is first out?"=w258:bool)
              n294 = property on="Status Out" class="Str"("Value"=w259) -> ()  [unwired: 2 in, 2 out]
              n295 = property on="first" class="Bool (strict)"("Value"=w258) -> ()  [unwired: 2 in, 2 out]
            }
            frame #4 {
              n296 = property on="first" class="Bool (strict)"() -> ("Value"=w268:bool)  [unwired: 2 in, 2 out]
              n297 = property on="Status Out" class="Str"() -> ("Value"=w270:string)  [unwired: 2 in, 2 out]
              n298 = property on="PH3?" class="Bool (strict)"() -> ("Value"=w271:bool)  [unwired: 2 in, 2 out]
              n299 = property on="PH3 Run" class="Bool (strict)"() -> ("Value"=w264:bool)  [unwired: 2 in, 2 out]
              n300 = property on="PH3 Prep" class="Bool (strict)"() -> ("Value"=w266:bool)  [unwired: 2 in, 2 out]
              n301 = call "flow_strings.vi"("string in"=w270, "is first in?"=w268, "use source?"=w271, "name"="PH3", "run source?"=w264, "prep source?"=w266, "is prep?"=w265) -> ("string out"=w269:string, "is first out?"=w267:bool)
              n302 = property on="Status Out" class="Str"("Value"=w269) -> ()  [unwired: 2 in, 2 out]
              n303 = property on="first" class="Bool (strict)"("Value"=w267) -> ()  [unwired: 2 in, 2 out]
            }
            frame #5 {
              n304 = property on="first" class="Bool (strict)"() -> ("Value"=w277:bool)  [unwired: 2 in, 2 out]
              n305 = property on="Status Out" class="Str"() -> ("Value"=w279:string)  [unwired: 2 in, 2 out]
              n306 = property on="AsH3?" class="Bool (strict)"() -> ("Value"=w280:bool)  [unwired: 2 in, 2 out]
              n307 = property on="AsH3 Run" class="Bool (strict)"() -> ("Value"=w273:bool)  [unwired: 2 in, 2 out]
              n308 = property on="AsH3 Prep" class="Bool (strict)"() -> ("Value"=w275:bool)  [unwired: 2 in, 2 out]
              n309 = call "flow_strings.vi"("string in"=w279, "is first in?"=w277, "use source?"=w280, "name"="AsH3", "run source?"=w273, "prep source?"=w275, "is prep?"=w274) -> ("string out"=w276:string, "is first out?"=w278:bool)
              n310 = property on="Status Out" class="Str"("Value"=w276) -> ()  [unwired: 2 in, 2 out]
              n311 = property on="first" class="Bool (strict)"("Value"=w278) -> ()  [unwired: 2 in, 2 out]
            }
            frame #6 {
              n312 = property on="Pbub?" class="Bool (strict)"() -> ("Value"=w282:bool)  [unwired: 2 in, 2 out]
              n313 = property on="first" class="Bool (strict)"() -> ("Value"=w287:bool)  [unwired: 2 in, 2 out]
              n314 = property on="Status Out" class="Str"() -> ("Value"=w289:string)  [unwired: 2 in, 2 out]
              n315 = property on="Pbub Run" class="Bool (strict)"() -> ("Value"=w283:bool)  [unwired: 2 in, 2 out]
              n316 = property on="Pbub Prep" class="Bool (strict)"() -> ("Value"=w284:bool)  [unwired: 2 in, 2 out]
              n317 = call "flow_strings.vi"("string in"=w289, "is first in?"=w287, "use source?"=w282, "name"="Pbub", "run source?"=w283, "prep source?"=w284, "is prep?"=w285) -> ("string out"=w288:string, "is first out?"=w286:bool)
              n318 = property on="Status Out" class="Str"("Value"=w288) -> ()  [unwired: 2 in, 2 out]
              n319 = property on="first" class="Bool (strict)"("Value"=w286) -> ()  [unwired: 2 in, 2 out]
            }
          }
        }
        frame #3 {
          n320 = local read "run started"() -> (w296:bool)
          n321 = local read "prep_done"() -> (w294:bool)
          n322 = Not(x=w296) -> (.not. x?=w297:bool)
          n323 = And(x=w294, y=w297) -> (x .and. y?=w295:bool)
          n324 = stacked-sequence {
            tunnel: w295 -> [w301]
            tunnel: w293 -> [w300]
            tunnel: w292 -> [w299]
            tunnel: [w298] -> w291
            frame #0 {
              n325 = case shown="True" w301 {
                tunnel: w300 -> [_ w305]
                tunnel: w299 -> [w302 w304]
                tunnel: [w302 w303] -> w298
                frame False {
                }
                frame True {
                  n326 = stacked-sequence {
                    tunnel: w305 -> [w306 w313 w323 w330 w337 w344 _]
                    tunnel: w304 -> [_ _ _ _ _ _ w352]
                    tunnel: [_ _ _ _ _ _ w351] -> w303
                    frame #0 {
                      n327 = case shown="False" w306 {
                        frame False {
                          n328 = property on="Al?" class="Bool (strict)"() -> ("Value"=w307:bool)  [unwired: 2 in, 2 out]
                          n329 = case shown="True" w307 {
                            frame False {
                              w308 = FALSE ("Al Active")
                              n330 = call "set_Al.vi"("ALMFC1"=0.0 ("Aluminum Flow"), "Remote"=w308, "Run"=w308, "Bubbler In"=w308, "Active"=w308) -> ()  [unwired: 5 out]
                            }
                            frame True {
                              w312 = TRUE ("Al Active")
                              n331 = property on="Al Flow" class="DigNum (strict)"() -> ("Value"=w311:dbl)  [unwired: 2 in, 2 out]
                              n332 = property on="Al Run" class="Bool (strict)"() -> ("Value"=w310:bool)  [unwired: 2 in, 2 out]
                              n333 = call "set_Al.vi"("ALMFC1"=w311, "Run"=w310, "Bubbler In"=w312, "Active"=w312) -> ()  [unwired: 1 in, 5 out]
                            }
                          }
                        }
                        frame True {
                        }
                      }
                    }
                    frame #1 {
                      n334 = case shown="False" w313 {
                        frame False {
                          n335 = property on="Ga?" class="Bool (strict)"() -> ("Value"=w314:bool)  [unwired: 2 in, 2 out]
                          n336 = case shown="True" w314 {
                            frame False {
                              w316 = FALSE ("Ga Active")
                              w315 = 0.0 ("Ga Flow 1")
                              n337 = call "set_Ga.vi"("Active"=w316, "GAMFC3"=w315, "GAMFC2"=w315, "GAMFC1"=w315, "Bubbler In"=w316, "H2 Dilute"=w316, "Run"=w316, "Remote"=w316) -> ()  [unwired: 8 out]
                            }
                            frame True {
                              w321 = TRUE ("Ga Active")
                              n338 = property on="GAMFC3 var" class="DigNum (strict)"() -> ("Value"=w317:dbl)  [unwired: 2 in, 2 out]
                              n339 = property on="Ga Dilution" class="Bool (strict)"() -> ("Value"=w320:bool)  [unwired: 2 in, 2 out]
                              n340 = property on="Ga Run" class="Bool (strict)"() -> ("Value"=w322:bool)  [unwired: 2 in, 2 out]
                              n341 = property on="GAMFC2 var" class="DigNum (strict)"() -> ("Value"=w318:dbl)  [unwired: 2 in, 2 out]
                              n342 = property on="GAMFC1 var" class="DigNum (strict)"() -> ("Value"=w319:dbl)  [unwired: 2 in, 2 out]
                              n343 = call "set_Ga.vi"("Active"=w321, "GAMFC3"=w317, "GAMFC2"=w318, "GAMFC1"=w319, "Bubbler In"=w321, "H2 Dilute"=w320, "Run"=w322, "Remote"=w321) -> ()  [unwired: 8 in]
                            }
                          }
                        }
                        frame True {
                        }
                      }
                    }
                    frame #2 {
                      n344 = case shown="False" w323 {
                        frame False {
                          n345 = property on="In?" class="Bool (strict)"() -> ("Value"=w324:bool)  [unwired: 2 in, 2 out]
                          n346 = case shown="True" w324 {
                            frame False {
                              w326 = FALSE ("In Remote")
                              n347 = call "set_In.vi"("INMFC1"=0.0 ("Indium Flow"), "Remote"=w326, "Run"=w326, "Bubbler In"=w326, "Active"=w326) -> ()  [unwired: 5 out]
                            }
                            frame True {
                              w329 = TRUE ("In Run")
                              n348 = property on="In Run" class="Bool (strict)"() -> ("Value"=w327:bool)  [unwired: 2 in, 2 out]
                              n349 = property on="In Flow" class="DigNum (strict)"() -> ("Value"=w328:dbl)  [unwired: 2 in, 2 out]
                              n350 = call "set_In.vi"("INMFC1"=w328, "Run"=w327, "Bubbler In"=w329, "Active"=w329) -> ()  [unwired: 1 in, 5 out]
                            }
                          }
                        }
                        frame True {
                        }
                      }
                    }
                    frame #3 {
                      n351 = case shown="False" w330 {
                        frame False {
                          n352 = property on="PH3?" class="Bool (strict)"() -> ("Value"=w331:bool)  [unwired: 2 in, 2 out]
                          n353 = case shown="True" w331 {
                            frame False {
                              w332 = FALSE ("P_Gas Active")
                              n354 = call "set_P_gas.vi"("Run"=w332, "Gas In"=w332, "Active"=w332, "P_Gas Remote"=w332, "H2 Flush"=w332, "P_Gas Flow"=0.0) -> ()
                            }
                            frame True {
                              w335 = TRUE ("P_Gas Active")
                              n355 = property on="PH3 Flow" class="DigNum (strict)"() -> ("Value"=w336:dbl)  [unwired: 2 in, 2 out]
                              n356 = property on="PH3 Run" class="Bool (strict)"() -> ("Value"=w334:bool)  [unwired: 2 in, 2 out]
                              n357 = call "set_P_gas.vi"("Run"=w334, "Gas In"=w335, "Active"=w335, "H2 Flush"=w335, "P_Gas Flow"=w336) -> ()  [unwired: 1 in]
                            }
                          }
                        }
                        frame True {
                        }
                      }
                    }
                    frame #4 {
                      n358 = case shown="False" w337 {
                        frame False {
                          n359 = property on="AsH3?" class="Bool (strict)"() -> ("Value"=w338:bool)  [unwired: 2 in, 2 out]
                          n360 = case shown="True" w338 {
                            frame False {
                              w339 = FALSE ("As_Gas Active")
                              n361 = call "set_As_gas.vi"("Active"=w339, "As_Gas Flow"=0.0, "Gas In"=w339, "H2 Flush"=w339, "Run"=w339, "Remote"=w339) -> ()  [unwired: 10 in]
                            }
                            frame True {
                              w342 = TRUE ("As_Gas Active")
                              n362 = property on="AsH3 Run" class="Bool (strict)"() -> ("Value"=w341:bool)  [unwired: 2 in, 2 out]
                              n363 = property on="AsH3 Flow" class="DigNum (strict)"() -> ("Value"=w343:dbl)  [unwired: 2 in, 2 out]
                              n364 = call "set_As_gas.vi"("Active"=w342, "As_Gas Flow"=w343, "Gas In"=w342, "Run"=w341) -> ()  [unwired: 12 in]
                            }
                          }
                        }
                        frame True {
                        }
                      }
                    }
                    frame #5 {
                      n365 = case shown="False" w344 {
                        frame False {
                          n366 = property on="Pbub?" class="Bool (strict)"() -> ("Value"=w345:bool)  [unwired: 2 in, 2 out]
                          n367 = case shown="True" w345 {
                            frame False {
                              w346 = FALSE ("P_Gas Active")
                              n368 = call "set_P_Liq.vi"("flow 1"=0.0 ("P_Gas Flow"), "Remote"=w346, "Run"=w346, "Bubbler In"=w346, "Active"=w346) -> ()  [unwired: 5 in]
                            }
                            frame True {
                              w350 = TRUE ("P_Gas Active")
                              n369 = property on="Pbub Flow" class="DigNum (strict)"() -> ("Value"=w349:dbl)  [unwired: 2 in, 2 out]
                              n370 = property on="Pbub Run" class="Bool (strict)"() -> ("Value"=w348:bool)  [unwired: 2 in, 2 out]
                              n371 = call "set_P_Liq.vi"("flow 1"=w349, "Run"=w348, "Bubbler In"=w350, "Active"=w350) -> ()  [unwired: 6 in]
                            }
                          }
                        }
                        frame True {
                        }
                      }
                    }
                    frame #6 {
                      n372 = call "Set_Argument.vi"("Enable"=TRUE, "Argument"="run_started", "Argument List In"=w352) -> ("Argument List Out"=w351:string[])
                    }
                  }
                }
              }
            }
          }
        }
      }
    }
    frame "End" {
    }
    frame "Idle" {
    }
  }
  "Argument List Out" <- w10
